vi "get Zoom Level.vi"(11 "Camera in":refnum<class "Camera.lvclass">) -> (3 "Zoom Level":T1)   [LabVIEW 2015, in "Camera.lvclass"]
uses:
  Camera.lvclass
  Zoom Level.ctl
  Camera.lvclass/Camera.ctl
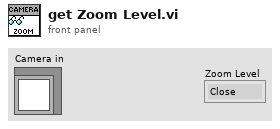
[diagram p1: front panel]
types:
  T1 = typedef "Camera.lvclass/Zoom Level.ctl" = enum16{"Close", "Medium", "Far"}
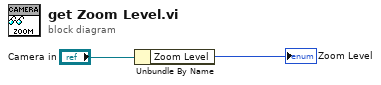
[diagram p0: block diagram]
diagram:
  n1 = Unbundle By Name("Camera in") -> ("Zoom Level"=→"Zoom Level":T1)
